vi "SafeParser_String.vi"(7 "Allowed Values":string[](array[string]), 9 "Array Index":i32, 11 "String Array":string[](array[string])) -> (0 "Error Out":errorcluster, 3 "Typecast Value":string)   [LabVIEW 2020]
doc: "This VI is configured for polymorphic use and takes in an array of strings and converts one of those strings (specified by an index) to a string. Error checking is performed including checking for acceptable data ranges. This VI is intended for use for the FRC 4265 autonomous parameter strings."
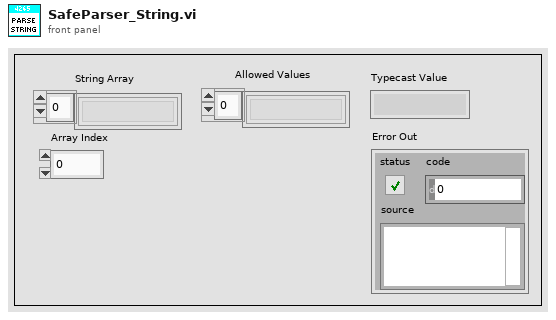
[diagram p1: front panel]
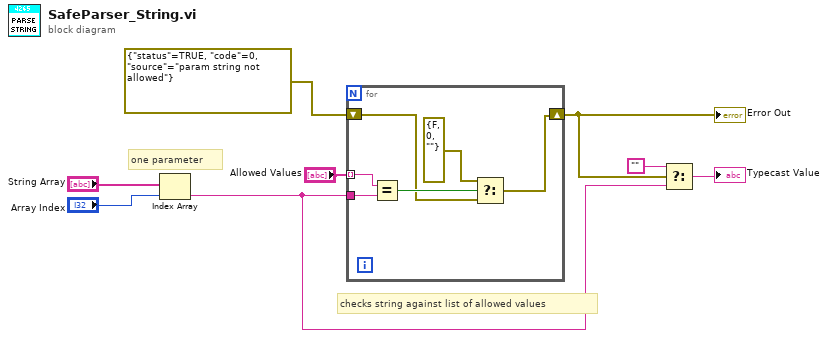
[diagram p0: block diagram]
diagram:
  # "checks string against list of allowed values"
  # "one parameter"
  n1 = Index Array(array="String Array", index="Array Index") -> (element=w2:string)
  n2 = for {
    tunnel: "Allowed Values" -> [w14] mode=indexing
    tunnel: w2 -> [w13]
    shift-right: [w10] -> w3
    shift-left: errorcluster {"status"=TRUE, "code"=0, "source"="param string not allowed"} ("error constant") -> [w11]
    n3 = Equal?(x=w14, y=w13) -> (x = y?=w12:bool)
    n4 = Select(t=errorcluster {"status"=FALSE, "code"=0, "source"=""} ("error constant"), s=w12, f=w11) -> (s? t:f=w10:errorcluster)
  }
  "Error Out" <- w3
  n5 = Select(t="", s=w3, f=w2) -> (s? t:f=→"Typecast Value":string)
